vi "Intan_Sampling_and_Streaming_Period.vi"(0 "VISA resource name":refnum<visa-resource-name>="COM1", 1 "error in":errorcluster, 2 "Desired Fs (Hz)":u16, 3 "Desired UART Stream Rate (Hz)":u16) -> (4 "VISA resource name out":refnum<visa-resource-name>, 5 "ADC_UART_Ratio":i32, 6 "FS actual (Hz)":i32, 7 "Actual Sampling Frequency (Hz)":string, 8 "error out":errorcluster)   [LabVIEW 2017]
doc: "use this VI to set the sampling rate (number samples/s/channel). Specify the rate in Hz. \nIn effect, this sets the intervalTimer object on the Teensyduino to precisely time ADC conversions. \nConversion time for 32 channels occurs in tens of microseconds typically. However, ther serial.write() commands typically take 2-6 ms, so the maximum sample rate expected is ~ 100 Hz."
panel:
  out "Stream Rate Request String":string
  out "ADC sample to Serial Sream Ratio":string
  out "UART stream rate written":string
  out "Coerced UART Stream Rate":u16
  in  "UART max (Hz)":u16=50
  in  "UART min (Hz)":u16
  out "Stream Rate  actual (Hz)":i32
  out "ack string":string
  out "Teensy fs string written":string
  in  "Teensy event char":string="m"
  # "ADC Sampilng"
  # "UART Streaming"
  # "Note: 50 Hz max streaming is empirical max stable rate for RN-42 bluetooth\n  Min value of 1 Hz is arbitrary.\n-JE Oct 26 2018"
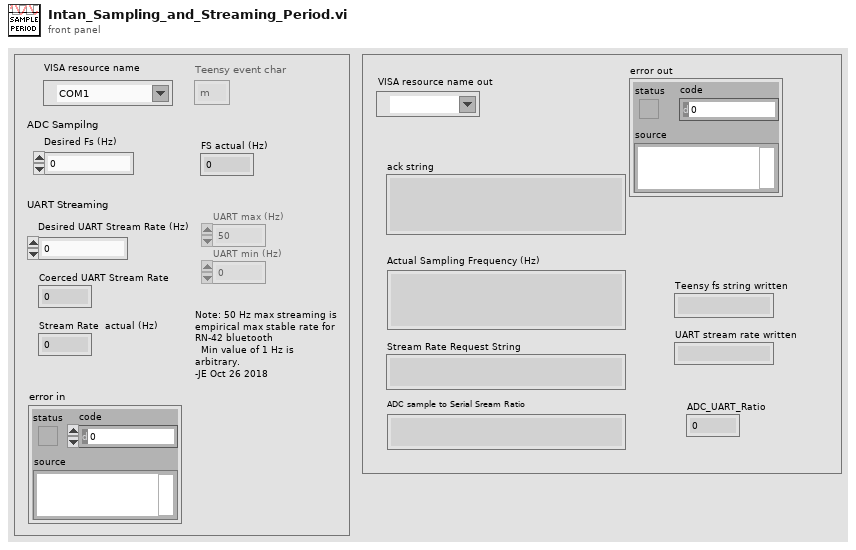
[diagram p1: front panel]
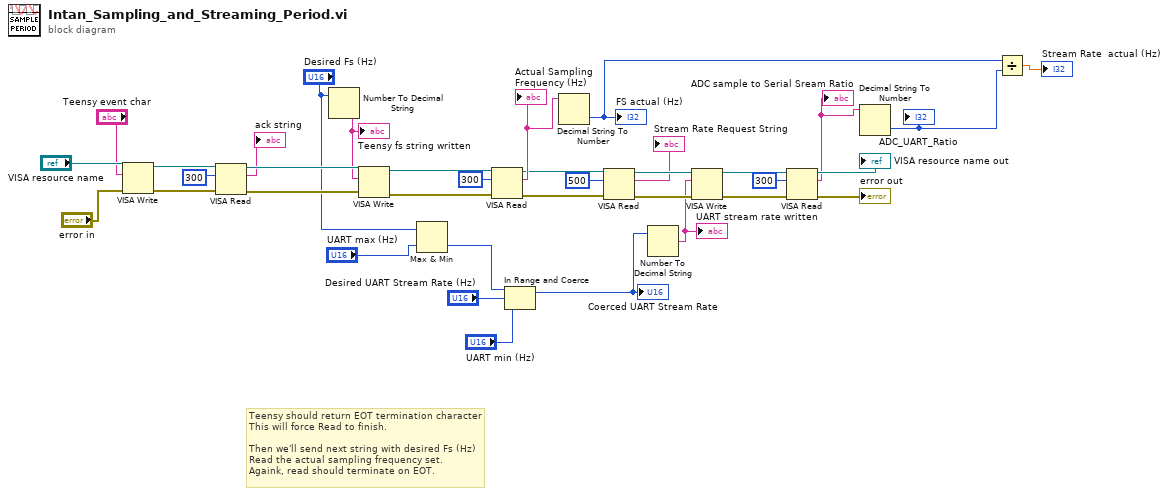
[diagram p0: block diagram]
diagram:
  # "Teensy should return EOT termination character \nThis will force Read to finish.\n\nThen we'll send next string with desired Fs (Hz)\nRead the actual sampling frequency set.\nAgaink, read should terminate on EOT."
  n1 = VISA Write(VISA resource name="VISA resource name", write buffer="Teensy event char", error in (no error)="error in") -> (VISA resource name out=w28:refnum<visa-resource-name>, error out=w27:errorcluster)  [unwired: 1 out]
  n2 = VISA Read(VISA resource name=w28, byte count=u32 300, error in (no error)=w27) -> (VISA resource name out=w34:refnum<visa-resource-name>, read buffer=→"ack string":string, error out=w33:errorcluster)  [unwired: 1 out]
  n3 = Number To Decimal String(number="Desired Fs (Hz)") -> (decimal integer string=w30:string)  [unwired: 1 in]
  "Teensy fs string written" <- w30
  n4 = VISA Write(VISA resource name=w34, write buffer=w30, error in (no error)=w33) -> (VISA resource name out=w25:refnum<visa-resource-name>, error out=w24:errorcluster)  [unwired: 1 out]
  n5 = Max & Min(x="Desired Fs (Hz)", y="UART max (Hz)") -> (min(x,y)=w4:u16)  [unwired: 1 out]
  n6 = VISA Read(VISA resource name=w25, byte count=u32 300, error in (no error)=w24) -> (VISA resource name out=w16:refnum<visa-resource-name>, read buffer=w29:string, error out=w19:errorcluster)  [unwired: 1 out]
  "Actual Sampling Frequency (Hz)" <- w29
  n7 = In Range and Coerce(upper limit=w4, x="Desired UART Stream Rate (Hz)", lower limit="UART min (Hz)") -> (coerced(x)=w13:u16)  [unwired: 1 out]
  "Coerced UART Stream Rate" <- w13
  n8 = Decimal String To Number(string=w29) -> (number=w1:i32)  [unwired: 2 in, 1 out]
  "FS actual (Hz)" <- w1
  n9 = VISA Read(VISA resource name=w16, byte count=u32 500, error in (no error)=w19) -> (VISA resource name out=w15:refnum<visa-resource-name>, read buffer=→"Stream Rate Request String":string, error out=w18:errorcluster)  [unwired: 1 out]
  n10 = Number To Decimal String(number=w13) -> (decimal integer string=w12:string)  [unwired: 1 in]
  "UART stream rate written" <- w12
  n11 = VISA Write(VISA resource name=w15, write buffer=w12, error in (no error)=w18) -> (VISA resource name out=w14:refnum<visa-resource-name>, error out=w17:errorcluster)  [unwired: 1 out]
  n12 = VISA Read(VISA resource name=w14, byte count=u32 300, error in (no error)=w17) -> (VISA resource name out=→"VISA resource name out":refnum<visa-resource-name>, read buffer=w8:string, error out=→"error out":errorcluster)  [unwired: 1 out]
  "ADC sample to Serial Sream Ratio" <- w8
  n13 = Decimal String To Number(string=w8) -> (number=w2:i32)  [unwired: 2 in, 1 out]
  "ADC_UART_Ratio" <- w2
  n14 = Divide(x=w1, y=w2) -> (x/y=→"Stream Rate  actual (Hz)":dbl)
